vi "build_AI_task.vi"(8 "error in":errorcluster caption="错误输入") -> (0 "error out":errorcluster caption="错误输出", 3 "task out":refnum<k21> caption="任务输出")   [LabVIEW 2013]
uses:
  <vilib>/DAQmx/create/channels.llb/DAQmx Create Channel (AI-Voltage-Basic).vi
  <vilib>/DAQmx/create/channels.llb/DAQmx Create Channel (TEDS-AI-Voltage-Basic).vi
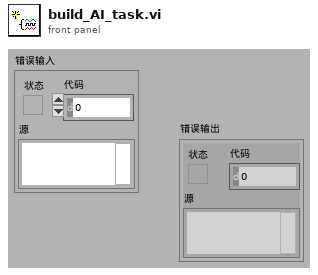
[diagram p1: front panel]
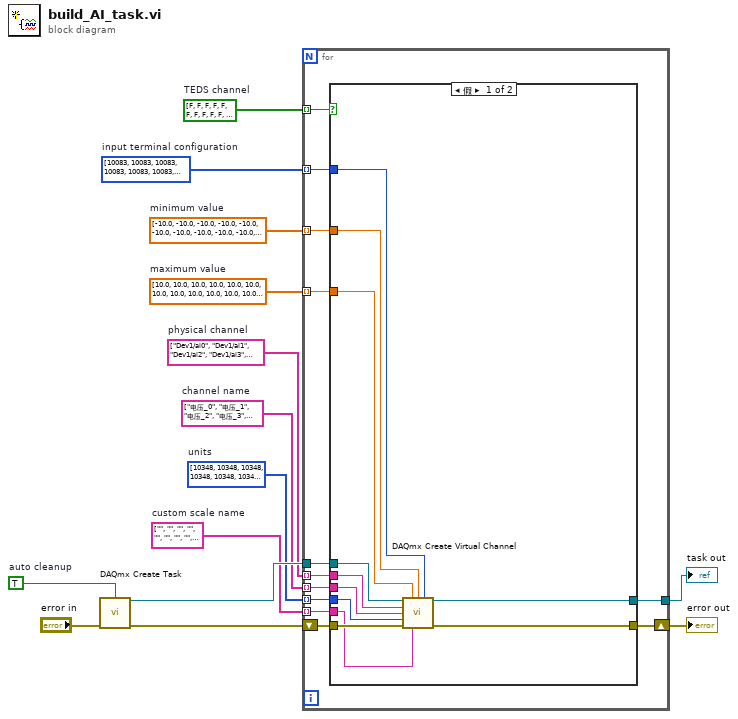
[diagram p0: block diagram]
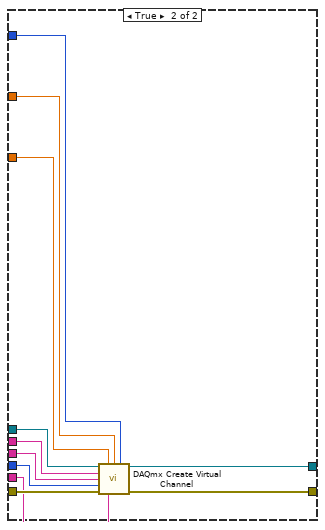
[diagram p2: hidden frame]
diagram:
  w1 = bool[] [FALSE, FALSE, FALSE, FALSE, FALSE, FALSE, FALSE, FALSE, FALSE, FALSE, FALSE, FALSE, FALSE, FALSE, FALSE, FALSE, FALSE, FALSE, FALSE, FALSE, FALSE, FALSE, FALSE, FALSE, FALSE, FALSE, FALSE, FALSE, FALSE, FALSE, FALSE, FALSE]  # TEDS channel
  w7 = string[] ["", "", "", "", "", "", "", "", "", "", "", "", "", "", "", "", "", "", "", "", "", "", "", "", "", "", "", "", "", "", "", ""]  # custom scale name
  w6 = i32[] [10348, 10348, 10348, 10348, 10348, 10348, 10348, 10348, 10348, 10348, 10348, 10348, 10348, 10348, 10348, 10348, 10348, 10348, 10348, 10348, 10348, 10348, 10348, 10348, 10348, 10348, 10348, 10348, 10348, 10348, 10348, 10348] items=["Volts"=10348, "From TEDS"=12516, "From Custom Scale"=10065]  # units
  w5 = string[] ["电压_0", "电压_1", "电压_2", "电压_3", "电压_4", "电压_5", "电压_6", "电压_7", "电压_8", "电压_9", "电压_10", "电压_11", "电压_12", "电压_13", "电压_14", "电压_15", "电压_16", "电压_17", "电压_18", "电压_19", "电压_20", "电压_21", "电压_22", "电压_23", "电压_24", "电压_25", "电压_26", "电压_27", "电压_28", "电压_29", "电压_30", "电压_31"]  # channel name
  w4 = string[] ["Dev1/ai0", "Dev1/ai1", "Dev1/ai2", "Dev1/ai3", "Dev1/ai4", "Dev1/ai5", "Dev1/ai6", "Dev1/ai7", "Dev1/ai8", "Dev1/ai9", "Dev1/ai10", "Dev1/ai11", "Dev1/ai12", "Dev1/ai13", "Dev1/ai14", "Dev1/ai15", "Dev1/ai16", "Dev1/ai17", "Dev1/ai18", "Dev1/ai19", "Dev1/ai20", "Dev1/ai21", "Dev1/ai22", "Dev1/ai23", "Dev1/ai24", "Dev1/ai25", "Dev1/ai26", "Dev1/ai27", "Dev1/ai28", "Dev1/ai29", "Dev1/ai30", "Dev1/ai31"]  # physical channel
  w8 = dbl[] [10.0, 10.0, 10.0, 10.0, 10.0, 10.0, 10.0, 10.0, 10.0, 10.0, 10.0, 10.0, 10.0, 10.0, 10.0, 10.0, 10.0, 10.0, 10.0, 10.0, 10.0, 10.0, 10.0, 10.0, 10.0, 10.0, 10.0, 10.0, 10.0, 10.0, 10.0, 10.0]  # maximum value
  w9 = dbl[] [-10.0, -10.0, -10.0, -10.0, -10.0, -10.0, -10.0, -10.0, -10.0, -10.0, -10.0, -10.0, -10.0, -10.0, -10.0, -10.0, -10.0, -10.0, -10.0, -10.0, -10.0, -10.0, -10.0, -10.0, -10.0, -10.0, -10.0, -10.0, -10.0, -10.0, -10.0, -10.0]  # minimum value
  w10 = i32[] [10083, 10083, 10083, 10083, 10083, 10083, 10083, 10083, 10083, 10083, 10083, 10083, 10083, 10083, 10083, 10083, 10083, 10083, 10083, 10083, 10083, 10083, 10083, 10083, 10083, 10083, 10083, 10083, 10083, 10083, 10083, 10083] items=["default"=-1, "RSE"=10083, "NRSE"=10078, "Differential"=10106, "Pseudodifferential"=12529]  # input terminal configuration
  w12 = TRUE  # auto cleanup
  n1 = call <vilib>:"DAQmx Create Task.vi"("auto cleanup"=w12, "error in"="error in") -> ("task out"=w11:refnum<k21>, "error out"=w13:errorcluster)  [unwired: 12 in]
  n2 = for "For循环" {
    tunnel: w11 -> [w23]
    tunnel: w10 -> [w24] mode=indexing
    tunnel: w9 -> [w25] mode=indexing
    tunnel: w8 -> [w26] mode=indexing
    tunnel: w7 -> [w16] mode=indexing
    tunnel: w6 -> [w17] mode=indexing
    tunnel: w5 -> [w19] mode=indexing
    tunnel: w4 -> [w18] mode=indexing
    tunnel: [w21] -> w3
    shift-right: [w20] -> w2
    shift-left: w13 -> [w22]
    tunnel: w1 -> [w15] mode=indexing
    n3 = case "条件结构" shown="假" w15 {
      tunnel: w26 -> [w37 w42]
      tunnel: w25 -> [w36 w43]
      tunnel: w24 -> [w35 w44]
      tunnel: w23 -> [w34 w48]
      tunnel: w22 -> [w33 w47]
      tunnel: [w32 w45] -> w21
      tunnel: [w31 w46] -> w20
      tunnel: w19 -> [w30 w40]
      tunnel: w18 -> [w29 w41]
      tunnel: w17 -> [w28 w39]
      tunnel: w16 -> [w27 w38]
      frame False {
        n4 = call-poly <vilib>:"DAQmx Create Virtual Channel.vi"("task in"=w34, "maximum value"=w37, "minimum value"=w36, "input terminal configuration"=w35, "physical channels"=w29, "name to assign"=w30, "units"=w28, "error in"=w33, "custom scale name"=w27) -> ("task out"=w32:refnum<k21>, "error out"=w31:errorcluster)  [unwired: 5 in]
      }
      frame True {
        n5 = call-poly <vilib>:"DAQmx Create Virtual Channel.vi"("task in"=w48, "maximum value"=w42, "minimum value"=w43, "input terminal configuration"=w44, "physical channels"=w41, "name to assign"=w40, "units"=w39, "error in"=w47, "custom scale name"=w38) -> ("task out"=w45:refnum<k21>, "error out"=w46:errorcluster)  [unwired: 5 in]
      }
    }
  }
  "error out" <- w2
  "task out" <- w3
